vi "RT_Act_Plant_v3 (SubVI).vi"(5 "Act_cmd (i-4) [rad]":dbl[](array[numeric]), 7 "Act_cmd (i-3) [rad]":dbl[](array[numeric]), 8 "Act_b(i-2)":dbl[](array[numeric]), 9 "Act_b(i-1)":dbl[](array[numeric]), 11 "Act_cmd (i-2) [rad]":dbl[](array[numeric])) -> (3 "Act_b":dbl[](array[numeric]))   [LabVIEW 2011]
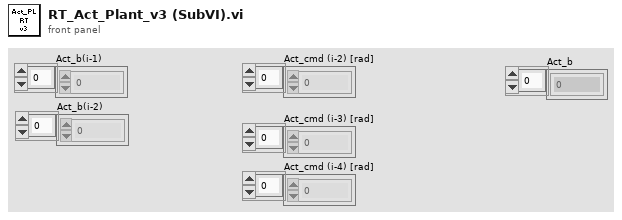
[diagram p1: front panel]
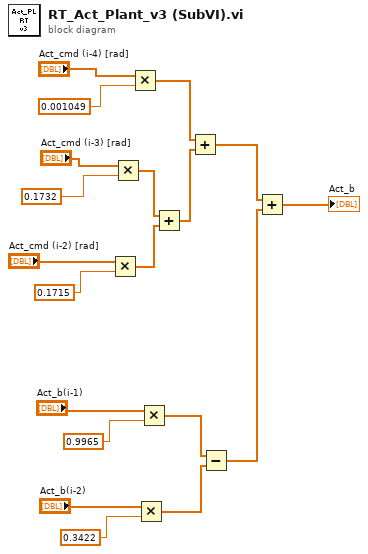
[diagram p0: block diagram]
diagram:
  n1 = Multiply(x="Act_cmd (i-2) [rad]", y=0.1715) -> (x*y=w9:dbl[])
  n2 = Multiply(x="Act_cmd (i-3) [rad]", y=0.1732) -> (x*y=w10:dbl[])
  n3 = Multiply(x="Act_cmd (i-4) [rad]", y=0.001049) -> (x*y=w3:dbl[])
  n4 = Multiply(x="Act_b(i-2)", y=0.3422) -> (x*y=w14:dbl[])
  n5 = Multiply(x="Act_b(i-1)", y=0.9965) -> (x*y=w15:dbl[])
  n6 = Add(x=w10, y=w9) -> (x+y=w2:dbl[])
  n7 = Add(x=w3, y=w2) -> (x+y=w1:dbl[])
  n8 = Subtract(x=w15, y=w14) -> (x-y=w8:dbl[])
  n9 = Add(x=w1, y=w8) -> (x+y=→"Act_b":dbl[])
